vi "IO Name to Enable Line.vi"(8 "error in (no error)":errorcluster, 10 "IO Name":string, 11 "RIO Target in":refnum<class "RIO Target.lvclass">) -> (0 "error out":errorcluster, 2 "Enable Line":string, 3 "RIO Target out":refnum<class "RIO Target.lvclass">)   [LabVIEW 2014, in "RIO Target.lvclass"]
uses:
  RIO Target.lvclass
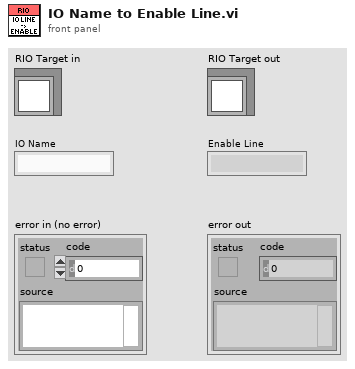
[diagram p1: front panel]
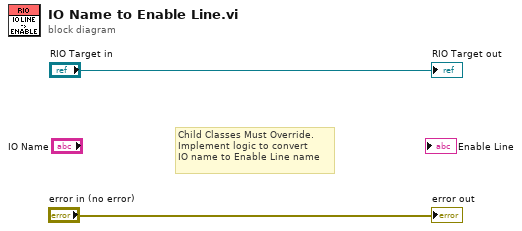
[diagram p0: block diagram]
diagram:
  # "Child Classes Must Override.\nImplement logic to convert \nIO name to Enable Line name"
  "error out" <- "error in (no error)"
  "RIO Target out" <- "RIO Target in"
